vi "_Update Start Up.vi"(4 "error in (no error)":errorcluster) -> (0 "error Out":errorcluster, 2 "Next InstrState":T1, 3 "Cancel":bool)   [LabVIEW 2018]
uses:
  Type/_RT Instrument State.ctl
  Type/_LCD Line1 Msg.ctl
  Type/_LCD Line2 Msg.ctl
  Type/_RT LED Num.ctl
  Type/_LED States.ctl
  Type/_RW Status.ctl
  _RT Global.vi
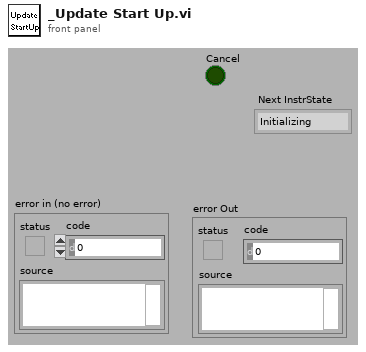
[diagram p1: front panel]
types:
  T1 = typedef "_RT Instrument State.ctl" = enum16{"Initializing", "Mass Spectrometer is Off", "Starting Up", "Turning Power Off", "Going to Standby", "Roughing Pump Ready", "Turning Turbo Off", "Turbo Startup", "Turbopump Ready", "Checking Vacuum", "Going to Ready", "Ready", "Running", "Source Standby", "Lost Communication", "Shutting Down", "Fault", "24V Standby", "Go to 24V Standby", "Turbopump Ready-Waiting"}
  T2 = typedef "_RT Startup Options.ctl" = cluster{"Door":bool, "Curtain":bool, "Pressure":bool, "Turbo":bool, "SysPoll":bool, "GasFlag":bool, "SourceExhaust":bool}
  T3 = typedef "_RT LED Num.ctl" = enum8{"ReadKey", "ClearKeyBuffer", "ClearLCD", "BacklightOn"}
  T4 = typedef "_LED States.ctl" = enum8{"Idle", "Solid B", "Solid R", "Solid P", "Off B", "Off R", "Off P", "Off BRP", "Off RP", "Flash R&P", "Flash P"}
  T5 = typedef "_RW Status.ctl" = enum8{"Done", "Do Read", "Do Write", "Set Latch1", "Set Latch2", "Set Latch3", "Set Latch4", "RP ON", "EL ON", "Serial Send", "Set LC Out", "Get LC In", "Read VAC", "Table Test", "Get Interlock", "Do Read2", "Do Write2"}
  T6 = typedef "_LCD Line2 Msg.ctl" = u16
  T7 = typedef "_LCD Line1 Msg.ctl" = u16
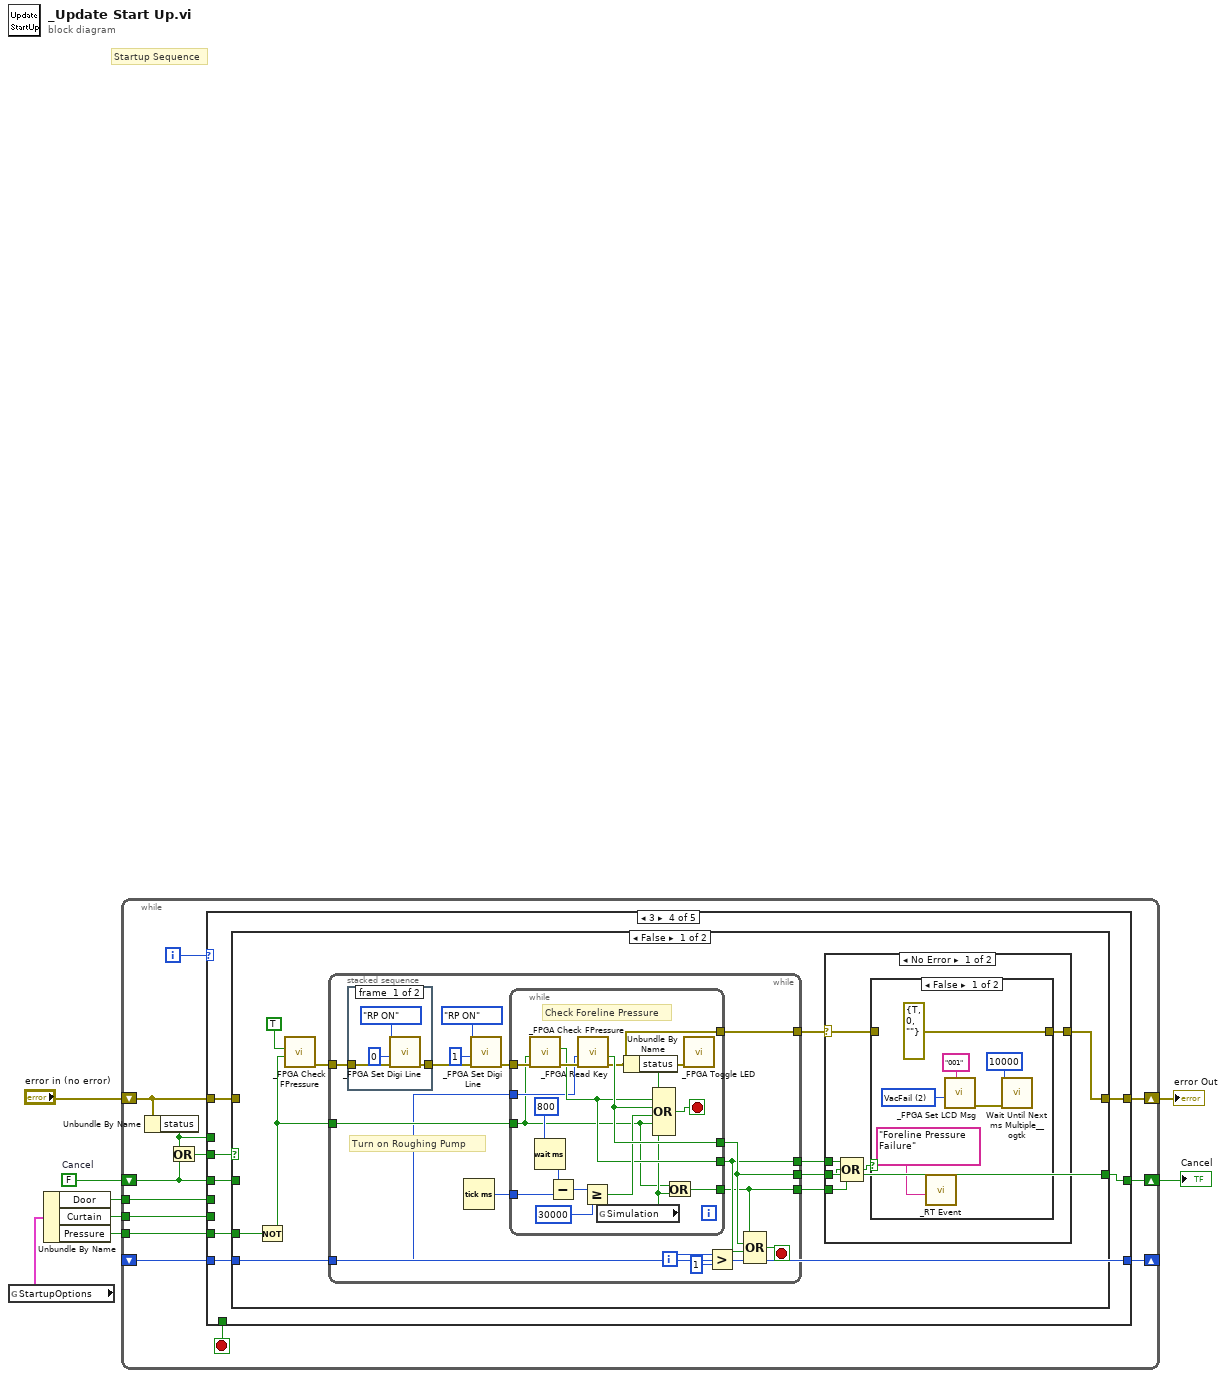
[diagram p0: block diagram]
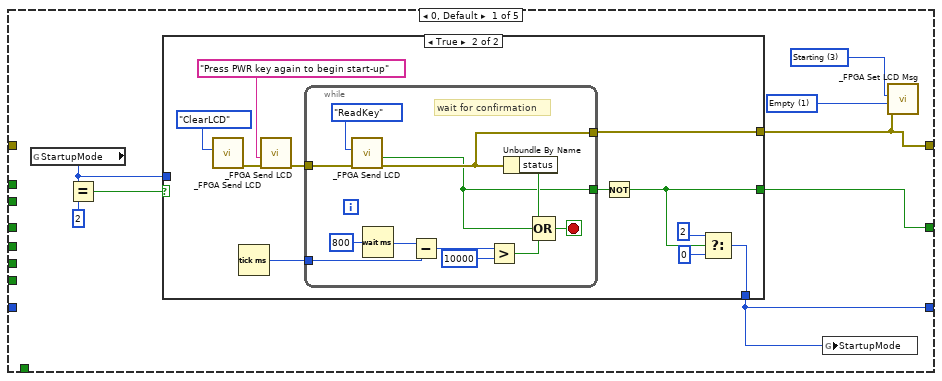
[diagram p2: hidden frame]
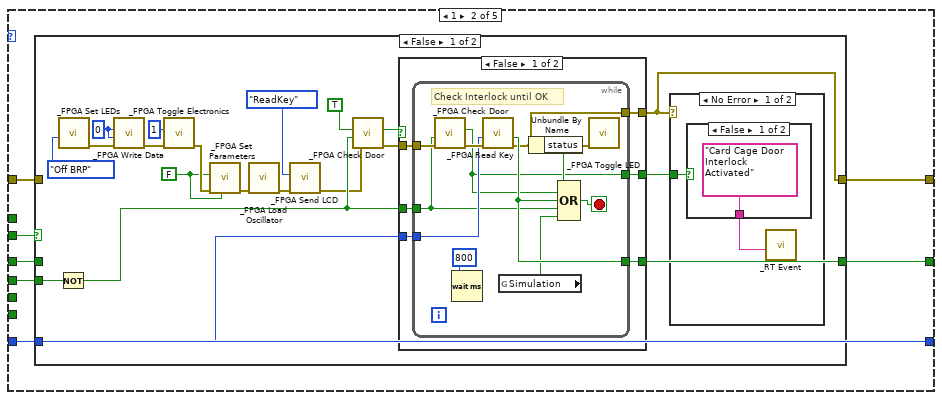
[diagram p4: hidden frame]
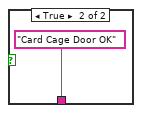
[diagram p6: hidden frame]
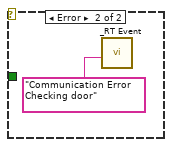
[diagram p7: hidden frame]
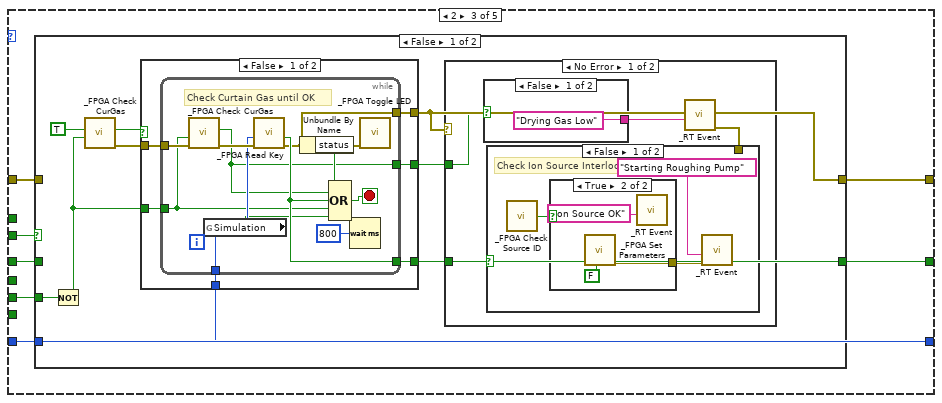
[diagram p9: hidden frame]
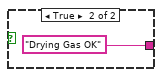
[diagram p13: hidden frame]
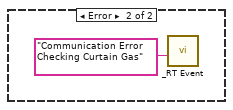
[diagram p14: hidden frame]
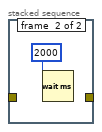
[diagram p16: hidden frame]
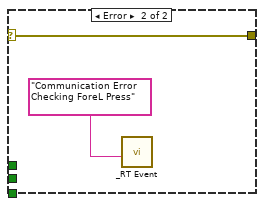
[diagram p18: hidden frame]
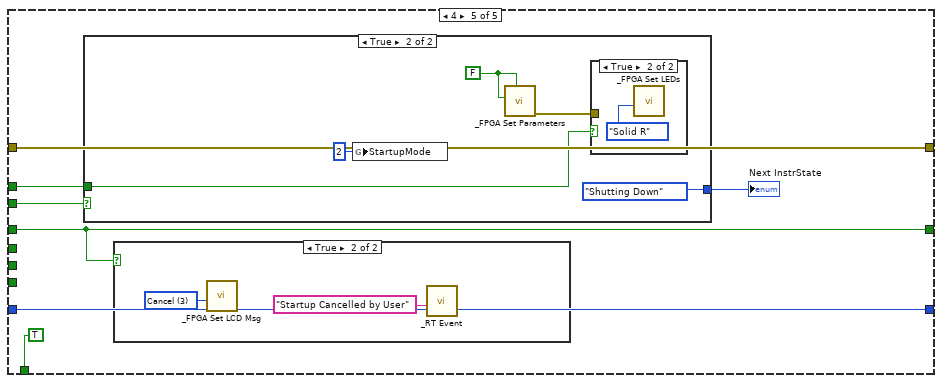
[diagram p20: hidden frame]
diagram:
  w7 = FALSE  # Cancel
  # "Startup Sequence"
  n1 = global read "_RT Global.vi" "StartupOptions"() -> (w4:T2)
  n2 = Unbundle By Name(w4) -> ("Door"=w3:bool, "Curtain"=w2:bool, "Pressure"=w1:bool)
  n3 = while {
    shift-right: [w17] -> w6
    shift-left: "error in (no error)" -> [w19]
    shift-right: [w16] -> w5
    shift-left: w7 -> [w18]
    tunnel: w3 -> [w9]
    tunnel: w2 -> [w14]
    tunnel: w1 -> [w13]
    shift-right: [w11] -> _
    shift-left: _ -> [w10]
    i -> [w21]
    stop <- w15 stop-if-true
    n4 = Unbundle By Name(w19) -> ("status"=w12:bool)
    n5 = Or(x=w12, y=w18) -> (x .or. y?=w20:bool)
    n6 = case shown="3" w21 {
      tunnel: w20 -> [_ w58 w111 w161 w232]
      tunnel: w19 -> [_ w57 w110 w160 w235]
      tunnel: w18 -> [_ w56 w109 w159 w233]
      tunnel: [w22 w60 w113 w163 w235] -> w17
      tunnel: [w27 w59 w112 w162 w233] -> w16
      tunnel: [_ _ _ _ TRUE] -> w15
      tunnel: w9 -> [_ w55 _ _ _]
      tunnel: w14 -> [_ _ w108 _ _]
      tunnel: w13 -> [_ _ _ w158 _]
      tunnel: w12 -> [_ _ _ _ w230]
      tunnel: [w25 w54 w107 w157 w229] -> w11
      tunnel: w10 -> [_ w54 w107 w157 w229]
      frame 0, Default {
        w24 = T6 1 items=["Same", "Empty", "VacFail", "Cancel", "CheckGas", "EleFail", "Probe1Fail", "Probe2Fail", "HeaterFail", "DoorOpen", "CheckComm", "PressStart"] ("Line2Msg (same)")
        w23 = T7 3 items=["Same", "Empty", "Connected", "Starting", "Stopping", "Action", "On", "Service", "Call", "Acquiring", "Source"] ("Line1Msg (same)")
        n7 = global read "_RT Global.vi" "StartupMode"() -> (w26:u8)
        n8 = Equal?(x=w26, y=u8 2) -> (x = y?=w28:bool)
        n9 = case shown="True" w28 {
          tunnel: [_ w40] -> w22
          tunnel: [_ w37] -> w27
          tunnel: [w30 w35] -> w25
          tunnel: w26 -> [w30 _]
          frame False {
          }
          frame True {
            n10 = call "_FPGA Send LCD.vi"("Command"=_RT_LED_Num."ClearLCD" ("LED#")) -> ("error out"=w34:errorcluster)  [unwired: 4 in, 3 out]
            n11 = Tick Count (ms)() -> (millisecond timer value=w41:u32)
            n12 = call "_FPGA Send LCD.vi"("error in (no error)"=w34, "Message"="Press PWR key again to begin start-up" ("Command")) -> ("error out"=w32:errorcluster)  [unwired: 3 in, 3 out]
            n13 = while {
              tunnel: w32 -> [w45]
              tunnel: [w44] -> w40
              tunnel: w41 -> [w49]
              tunnel: [w42] -> w39
              stop <- w52 stop-if-true
              # "wait for confirmation"
              n14 = call "_FPGA Send LCD.vi"("error in (no error)"=w45, "Command"=_RT_LED_Num."ReadKey" ("LED#")) -> ("error out"=w44:errorcluster, "Key Pressed"=w42:bool)  [unwired: 3 in, 2 out]
              n15 = Wait (ms)(milliseconds to wait=u32 800) -> (millisecond timer value=w50:u32)
              n16 = Subtract(x=w50, y=w49) -> (x-y=w48:u32)
              n17 = Greater?(x=w48, y=u32 10000) -> (0:w43:bool)
              n18 = Unbundle By Name(w44) -> ("status"=w51:bool)
              n19 = Compound Arithmetic op=OR(w51, w42, w43) -> (w52:bool)
            }
            n20 = Not(x=w39) -> (.not. x?=w37:bool)
            n21 = Select(t=u8 2 ("f"), s=w37, f=u8 0) -> (s? t:f=w35:u8)
          }
        }
        n22 = global write "_RT Global.vi" "StartupMode"(w25) -> ()
        n23 = call "_FPGA Set LCD Msg.vi"("error in"=w22, "Line2Msg (same)"=w24, "Line1Msg (same)"=w23) -> ()  [unwired: 4 in, 3 out]
      }
      frame 1 {
        n24 = case shown="False" w58 {
          tunnel: [w64 w105] -> w59
          tunnel: [w63 w106] -> w60
          tunnel: w57 -> [_ w106]
          tunnel: w56 -> [_ w105]
          tunnel: w55 -> [w65 _]
          tunnel: w54 -> [w68 _]
          frame False {
            w70 = FALSE ("HSID Temp (on)")
            w78 = u16 0 ("Address")
            n25 = Not(x=w65) -> (.not. x?=w62:bool)
            n26 = call "_FPGA Set LEDs.vi"("LED Command"=_LED_States."Off BRP") -> ("error out"=w76:errorcluster)  [unwired: 3 in, 3 out]
            n27 = call "_FPGA Write Data.vi"("error in"=w76, "Data"=w78, "Address"=w78) -> ("error out"=w77:errorcluster)  [unwired: 3 in, 2 out]
            n28 = call "_FPGA Toggle Electronics.vi"("error in"=w77, "Ele On (1 for ON and 0 for OFF)"=u32 1 ("States")) -> ("error out"=w75:errorcluster)  [unwired: 1 in, 5 out]
            n29 = call "_FPGA Set Parameters.vi"("ExhaustGas (on)"=w70, "error in"=w75, "HSID Temp (on)"=w70) -> ("error out"=w71:errorcluster)  [unwired: 6 in, 2 out]
            n30 = call "_FPGA Load Oscillator.vi"("error in"=w71) -> ("error out"=w66:errorcluster)  [unwired: 2 in, 4 out]
            n31 = call "_FPGA Send LCD.vi"("error in (no error)"=w66, "Command"=_RT_LED_Num."ReadKey" ("LED#")) -> ("error out"=w61:errorcluster)  [unwired: 3 in, 3 out]
            n32 = call "_FPGA Check Door.vi"("error in"=w61, "DisableCheck (F)"=w62, "CheckNow (F)"=TRUE) -> ("error out"=w74:errorcluster, "DoorOK"=w72:bool)  [unwired: 1 in, 2 out]
            n33 = case shown="False" w72 {
              selector: w72 -> [_ w98]
              tunnel: [w86 _] -> w64
              tunnel: [w85 w99] -> w63
              tunnel: w74 -> [w84 w99]
              tunnel: w62 -> [w83 _]
              tunnel: w68 -> [w82 _]
              tunnel: [w81 w98] -> w69
              frame False {
                n34 = while {
                  tunnel: w84 -> [w96]
                  tunnel: [w87] -> w85
                  tunnel: [w91] -> w86
                  tunnel: w83 -> [w88]
                  tunnel: w82 -> [w93]
                  tunnel: [w89] -> w81
                  stop <- w92 stop-if-true
                  # "Check Interlock until OK"
                  n35 = call "_FPGA Check Door.vi"("error in"=w96, "DisableCheck (F)"=w88) -> ("error out"=w94:errorcluster, "DoorOK"=w89:bool)  [unwired: 2 in, 2 out]
                  n36 = Wait (ms)(milliseconds to wait=u32 800) -> ()  [unwired: 1 out]
                  n37 = call "_FPGA Read Key.vi"("error in (no error)"=w94, "CurStartupMode (0)"=w93) -> ("error out"=w87:errorcluster, "Key Pressed"=w91:bool)  [unwired: 2 in, 3 out]
                  n38 = global read "_RT Global.vi" "Simulation"() -> (w90:bool)
                  n39 = Unbundle By Name(w87) -> ("status"=w97:bool)
                  n40 = Compound Arithmetic op=OR(w97, w89, w91, w88, w90) -> (w92:bool)
                  n41 = call "_FPGA Toggle LED.vi"("error in (no error)"=w87) -> ()  [unwired: 4 in, 4 out]
                }
              }
              frame True {
              }
            }
            n42 = case shown="No Error" w63 {
              tunnel: w69 -> [w101 _]
              frame No Error {
                n43 = case shown="False" w101 {
                  tunnel: ["Card Cage Door Interlock Activated" "Card Cage Door OK"] -> w100
                  frame False {
                  }
                  frame True {
                  }
                }
                n44 = call "_RT Event.vi"("Event"=w100) -> ()  [unwired: 2 in, 5 out]
              }
              frame Error {
                n45 = call "_RT Event.vi"("Event"="Communication Error Checking door") -> ()  [unwired: 2 in, 5 out]
              }
            }
          }
          frame True {
          }
        }
      }
      frame 2 {
        n46 = case shown="False" w111 {
          tunnel: [w117 w155] -> w112
          tunnel: [w122 w156] -> w113
          tunnel: w110 -> [_ w156]
          tunnel: w109 -> [_ w155]
          tunnel: w108 -> [w118 _]
          tunnel: w107 -> [w115 _]
          frame False {
            n47 = Not(x=w118) -> (.not. x?=w114:bool)
            n48 = call "_FPGA Check CurGas.vi"("DisableCheck (F)"=w114, "CheckNow (F)"=TRUE) -> ("error out"=w121:errorcluster, "CurGasOK"=w119:bool)  [unwired: 3 in, 1 out]
            n49 = case shown="False" w119 {
              selector: w119 -> [_ w140]
              tunnel: [w128 _] -> w117
              tunnel: [w127 w141] -> w122
              tunnel: w121 -> [w126 w141]
              tunnel: w114 -> [w125 _]
              tunnel: w115 -> [w124 _]
              tunnel: [w123 w140] -> w116
              frame False {
                n50 = while {
                  tunnel: w126 -> [w135]
                  tunnel: [w129] -> w127
                  tunnel: [w136] -> w128
                  tunnel: w125 -> [w130]
                  tunnel: w124 -> [w133]
                  tunnel: [w132] -> w123
                  stop <- w139 stop-if-true
                  # "Check Curtain Gas until OK"
                  n51 = call "_FPGA Check CurGas.vi"("error in"=w135, "DisableCheck (F)"=w130) -> ("error out"=w134:errorcluster, "CurGasOK"=w132:bool)  [unwired: 3 in, 1 out]
                  n52 = global read "_RT Global.vi" "Simulation"() -> (w131:bool)
                  n53 = call "_FPGA Read Key.vi"("error in (no error)"=w134, "CurStartupMode (0)"=w133) -> ("error out"=w129:errorcluster, "Key Pressed"=w136:bool)  [unwired: 2 in, 3 out]
                  n54 = Unbundle By Name(w129) -> ("status"=w138:bool)
                  n55 = Compound Arithmetic op=OR(w138, w132, w136, w130, w131) -> (w139:bool)
                  n56 = Wait (ms)(milliseconds to wait=u32 800) -> ()  [unwired: 1 out]
                  n57 = call "_FPGA Toggle LED.vi"("error in (no error)"=w129) -> ()  [unwired: 3 in, 5 out]
                }
              }
              frame True {
              }
            }
            n58 = case shown="No Error" w122 {
              tunnel: w117 -> [w144 _]
              tunnel: w116 -> [w145 _]
              frame No Error {
                n59 = case shown="False" w145 {
                  tunnel: ["Drying Gas Low" "Drying Gas OK"] -> w142
                  frame False {
                  }
                  frame True {
                  }
                }
                n60 = call "_RT Event.vi"("Event"=w142) -> ("error out"=w143:errorcluster)  [unwired: 2 in, 4 out]
                n61 = case shown="False" w144 {
                  tunnel: w143 -> [_ _]
                  frame False {
                    # "Check Ion Source Interlock"
                    n62 = call "_FPGA Check Source ID.vi"() -> ("Source ID OK"=w148:bool)  [unwired: 1 in]
                    n63 = case shown="True" w148 {
                      tunnel: [_ w150] -> w147
                      frame False {
                      }
                      frame True {
                        n64 = call "_FPGA Set Parameters.vi"("ExhaustGas (on)"=FALSE) -> ("error out"=w150:errorcluster)  [unwired: 8 in, 2 out]
                        n65 = call "_RT Event.vi"("Event"="Ion Source OK") -> ()  [unwired: 2 in, 5 out]
                      }
                    }
                    n66 = call "_RT Event.vi"("error in (no error)"=w147, "Event"="Starting Roughing Pump") -> ()  [unwired: 1 in, 5 out]
                  }
                  frame True {
                  }
                }
              }
              frame Error {
                n67 = call "_RT Event.vi"("Event"="Communication Error Checking Curtain Gas") -> ()  [unwired: 2 in, 5 out]
              }
            }
          }
          frame True {
          }
        }
      }
      frame 3 {
        n68 = case shown="False" w161 {
          tunnel: [w169 w227] -> w162
          tunnel: [w171 w228] -> w163
          tunnel: w160 -> [_ w228]
          tunnel: w159 -> [_ w227]
          tunnel: w158 -> [w170 _]
          tunnel: w157 -> [w165 _]
          frame False {
            n69 = Not(x=w170) -> (.not. x?=w164:bool)
            n70 = call "_FPGA Check FPressure.vi"("DisableCheck (F)"=w164, "CheckNow (F)"=TRUE) -> ("error out"=w167:errorcluster)  [unwired: 3 in, 2 out]
            n71 = while {
              tunnel: [w184] -> w173
              tunnel: [w183] -> w169
              tunnel: [w182] -> w172
              tunnel: w164 -> [w181]
              tunnel: w167 -> [w177]
              tunnel: [w175] -> w166
              tunnel: w165 -> [w174]
              i -> [w188]
              stop <- w186 stop-if-true
              # "Turn on Roughing Pump"
              n72 = stacked-sequence {
                tunnel: w177 -> [w191 _]
                tunnel: [w190 _] -> w178
                frame #0 {
                  n73 = call "_FPGA Set Digi Line.vi"("error in"=w191, "States"=u16 0, "Line (Set Latch1)"=_RW_Status."RP ON") -> ("error out"=w190:errorcluster)  [unwired: 1 in, 3 out]
                }
                frame #1 {
                  n74 = Wait (ms)(milliseconds to wait=u32 2000) -> ()  [unwired: 1 out]
                }
              }
              n75 = Tick Count (ms)() -> (millisecond timer value=w185:u32)
              n76 = call "_FPGA Set Digi Line.vi"("error in"=w178, "States"=u16 1, "Line (Set Latch1)"=_RW_Status."RP ON") -> ("error out"=w176:errorcluster)  [unwired: 1 in, 3 out]
              n77 = while {
                tunnel: w176 -> [w207]
                tunnel: [w195] -> w184
                tunnel: [w208] -> w183
                tunnel: w185 -> [w202]
                tunnel: [w200] -> w182
                tunnel: w181 -> [w196]
                tunnel: w174 -> [w199]
                tunnel: [w197] -> w175
                stop <- w211 stop-if-true
                # "Check Foreline Pressure"
                n78 = call "_FPGA Check FPressure.vi"("error in"=w207, "DisableCheck (F)"=w196) -> ("error out"=w206:errorcluster, "PressureOK"=w200:bool)  [unwired: 2 in, 2 out]
                n79 = Wait (ms)(milliseconds to wait=u32 800) -> (millisecond timer value=w203:u32)
                n80 = Subtract(x=w203, y=w202) -> (x-y=w204:u32)
                n81 = call "_FPGA Read Key.vi"("error in (no error)"=w206, "CurStartupMode (0)"=w199) -> ("error out"=w195:errorcluster, "Key Pressed"=w208:bool)  [unwired: 2 in, 3 out]
                n82 = Greater Or Equal?(x=w204, y=u32 30000) -> (x >= y?=w201:bool)
                n83 = global read "_RT Global.vi" "Simulation"() -> (w198:bool)
                n84 = Unbundle By Name(w195) -> ("status"=w210:bool)
                n85 = Compound Arithmetic op=OR(w210, w200, w208, w201, w196, w198) -> (w211:bool)
                n86 = Or(x=w196, y=w198) -> (x .or. y?=w197:bool)
                n87 = call "_FPGA Toggle LED.vi"("error in (no error)"=w195) -> ()  [unwired: 4 in, 4 out]
              }
              n88 = Greater?(x=w188, y=1) -> (0:w187:bool)
              n89 = Compound Arithmetic op=OR(w175, w183, w182, w187) -> (w186:bool)
            }
            n90 = case shown="No Error" w173 {
              selector: w173 -> [w217 w226]
              tunnel: w172 -> [w214 _]
              tunnel: [w216 w226] -> w171
              tunnel: w166 -> [w213 _]
              tunnel: w169 -> [w212 _]
              frame No Error {
                n91 = Compound Arithmetic op=OR(w214, w212, w213) -> (w215:bool)
                n92 = case shown="False" w215 {
                  tunnel: w217 -> [_ w224]
                  tunnel: [errorcluster {"status"=TRUE, "code"=0, "source"=""} ("error IO") w224] -> w216
                  frame False {
                    w222 = T6 2 items=["Same", "Empty", "VacFail", "Cancel", "CheckGas", "EleFail", "Probe1Fail", "Probe2Fail", "HeaterFail", "DoorOpen", "CheckComm", "PressStart", "StartRP"] ("Line2Msg (same)")
                    n93 = call "_RT Event.vi"("Event"="Foreline Pressure   Failure" ("Command")) -> ()  [unwired: 2 in, 5 out]
                    n94 = call "_FPGA Set LCD Msg.vi"("ErrNum"="001", "Line2Msg (same)"=w222) -> ("error out"=w219:errorcluster)  [unwired: 5 in, 2 out]
                    n95 = call <userlib>:"Wait Until Next ms Multiple__ogtk.vi"("error in (no error)"=w219, "milliseconds to wait"=u32 10000) -> ()  [unwired: 8 in, 2 out]
                  }
                  frame True {
                  }
                }
              }
              frame Error {
                n96 = call "_RT Event.vi"("Event"="Communication Error Checking ForeL Press") -> ()  [unwired: 2 in, 5 out]
              }
            }
          }
          frame True {
          }
        }
      }
      frame 4 {
        n97 = case shown="True" w232 {
          tunnel: [_RT_Instrument_State."Roughing Pump Ready" ("Next InstrState") _RT_Instrument_State."Shutting Down" ("Next InstrState")] -> w231
          tunnel: w230 -> [_ w242]
          frame False {
            n98 = call "_RT Event.vi"("Event"="Roughing Pump OK" ("Command")) -> ()  [unwired: 2 in, 5 out]
          }
          frame True {
            w241 = FALSE
            n99 = global write "_RT Global.vi" "StartupMode"(u8 2 ("StartupMode")) -> ()
            n100 = call "_FPGA Set Parameters.vi"("ExhaustGas (on)"=w241, "CurGas (on)"=w241, "HSID Temp (on)"=w241) -> ("error out"=w238:errorcluster)  [unwired: 6 in, 2 out]
            n101 = case shown="True" w242 {
              tunnel: w238 -> [_ _]
              frame False {
              }
              frame True {
                n102 = call "_FPGA Set LEDs.vi"("LED Command"=_LED_States."Solid R") -> ()  [unwired: 3 in, 4 out]
              }
            }
          }
        }
        "Next InstrState" <- w231
        n103 = case shown="True" w233 {
          frame False {
          }
          frame True {
            w245 = T6 3 items=["Same", "Empty", "VacFail", "Cancel", "CheckGas", "EleFail", "Probe1Fail", "Probe2Fail", "HeaterFail", "DoorOpen", "CheckComm", "PressStart", "StartRP"] ("Line2Msg (same)")
            n104 = call "_FPGA Set LCD Msg.vi"("Line2Msg (same)"=w245) -> ()  [unwired: 6 in, 3 out]
            n105 = call "_RT Event.vi"("Event"="Startup Cancelled by User" ("Command")) -> ()  [unwired: 2 in, 5 out]
          }
        }
      }
    }
  }
  "error Out" <- w6
  "Cancel" <- w5
